vi "User scan tool box.vi"() -> ()   [LabVIEW 2021]
doc: "This example demonstrates how you can create your own \"toolbox\": a custom designed VI that regroups all the controls you want to access quickly.\n\nThis example displays the most used controls to perform STM scanning (current, bias, gain, scan frame, tilt).\n\n- Nanonis Programming Interface -"
uses:
  Nanonis Prog Interface.lvlib
panel:
  out "Status":bool
  in  "stop":bool
  in  "Bias (V)":sgl=0.5 min=-10 max=10 format="%_4p"
  in  "Speed":sgl(slide)=1.0 caption="Time per line (s)" min=0.01 max=10 scale=0.01..2.0 scale format="%.0p"
  in  "Current (A)":sgl=1e-09 format="%_4p"
  in  "Scan":bool
  in  "Images basename":string="SampleTest_"
  in  "Tilt Y (deg)":sgl min=-30 max=30 format="%.3f"
  in  "Tilt X (deg)":sgl min=-30 max=30 format="%.3f"
  in  "Position Yc":sgl min=-1e-05 max=1e-05 format="%.2p"
  in  "Position Xc":sgl min=-1e-05 max=1e-05 format="%.2p"
  in  "Height (m)":sgl=1e-07 min=1e-12 max=1e-05 format="%#.2p"
  in  "Width (m)":sgl=1e-07 min=1e-12 max=1e-05 format="%#.2p"
  in  "Angle (deg)":sgl format="%.2f"
  in  "P-gain":sgl(slide)=1e-10 scale=1e-11..1e-08 scale format="%.0p"
  in  "Lines":i32=256 min=1 max=2048
  in  "Pixels":i32=256 min=16 max=2048
  # "Scan parameters"
  # "Scan frame"
  # "Correction"
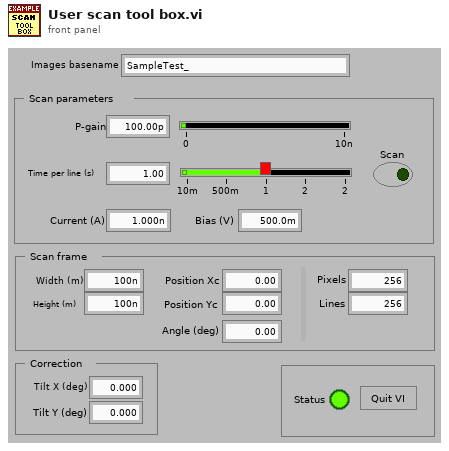
[diagram p1: front panel]
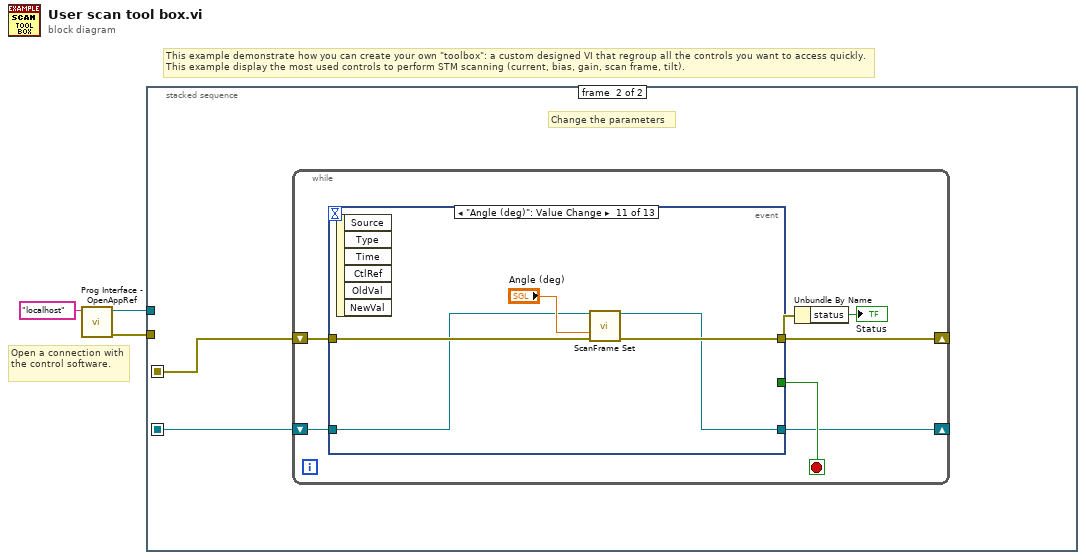
[diagram p0: block diagram]
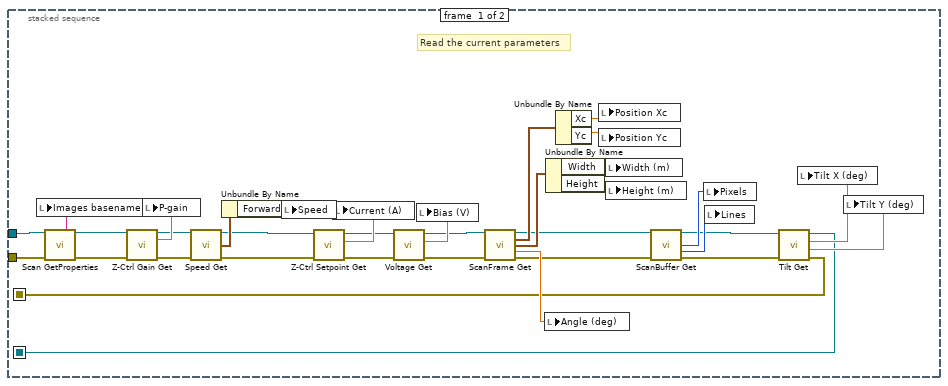
[diagram p2: hidden frame]
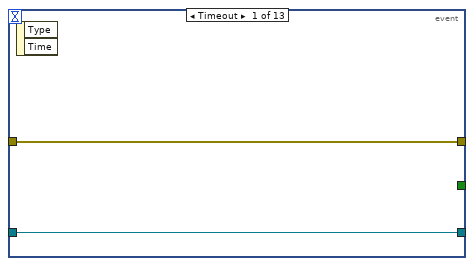
[diagram p3: hidden frame]
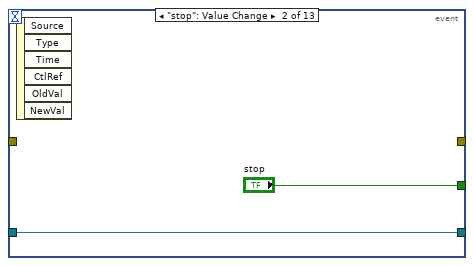
[diagram p4: hidden frame]
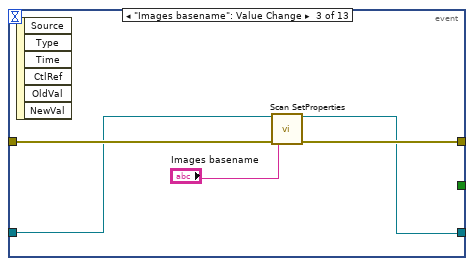
[diagram p5: hidden frame]
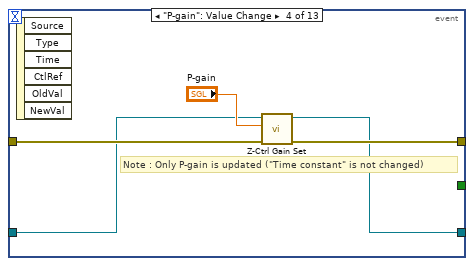
[diagram p6: hidden frame]
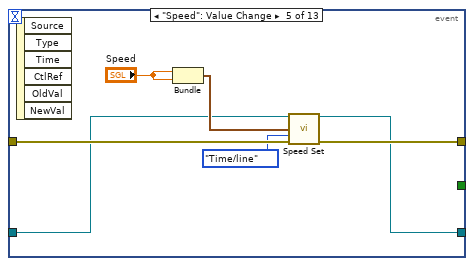
[diagram p7: hidden frame]
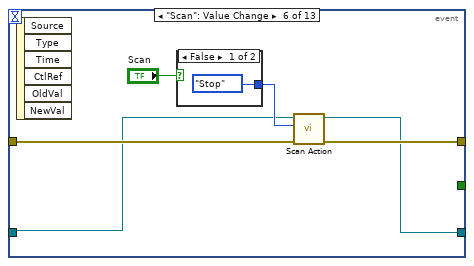
[diagram p8: hidden frame]
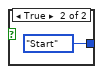
[diagram p9: hidden frame]
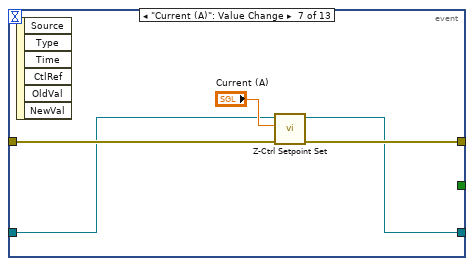
[diagram p10: hidden frame]
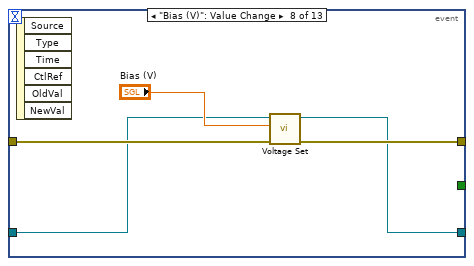
[diagram p11: hidden frame]
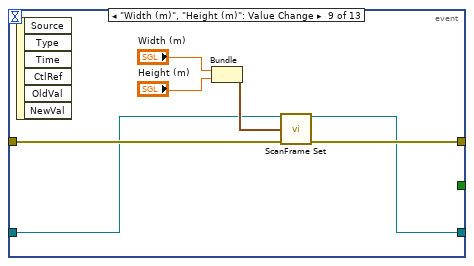
[diagram p12: hidden frame]
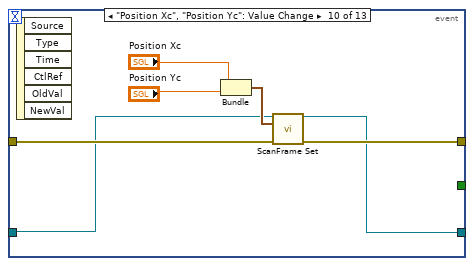
[diagram p13: hidden frame]
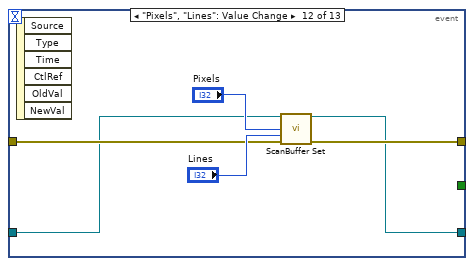
[diagram p14: hidden frame]
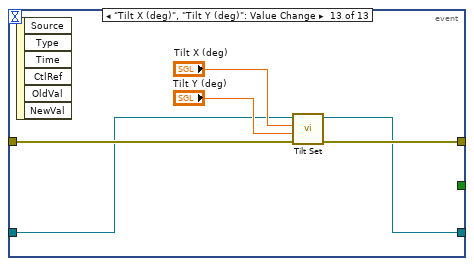
[diagram p15: hidden frame]
diagram:
  # "Open a connection with the control software."
  # "This example demonstrate how you can create your own \"toolbox\": a custom designed VI that regroup all the controls you want to access quickly.\nThis example display the most used controls to perform STM scanning (current, bias, gain, scan frame, tilt)."
  n1 = call <userlib>:"Prog Interface - OpenAppRef.vi"("Machine name (local machine IP)"="localhost" ("Machine name (localhost)")) -> ("Error out"=w2:errorcluster, "Application reference"=w1:refnum<vi>)  [unwired: 5 in]
  n2 = stacked-sequence {
    seq-local: [w19 _] -> [_ w40]
    seq-local: [w4 _] -> [_ w39]
    tunnel: w2 -> [w18 _]
    tunnel: w1 -> [w15 _]
    frame #0 {
      # "Read the current parameters"
      n3 = call <userlib>:"Scan GetProperties.vi"("Application ref in"=w15, "Error in (no error)"=w18) -> ("Application ref out"=w14:refnum<vi>, "Serie name"=w16:string, "Error out"=w17:errorcluster)  [unwired: 6 in, 5 out]
      n4 = local write "Images basename"(w16) -> ()
      n5 = call <userlib>:"Z-Ctrl Gain Get.vi"("Application ref in"=w14, "error in (no error)"=w17) -> ("Application ref out"=w13:refnum<vi>, "P-gain"=w38:sgl, "error out"=w37:errorcluster)  [unwired: 9 in, 2 out]
      n6 = local write "P-gain"(w38) -> ()
      n7 = call <userlib>:"Speed Get.vi"("Application ref in"=w13, "error in (no error)"=w37) -> ("Application ref out"=w12:refnum<vi>, "Time/line (s)"=w36:cluster{"Forward":sgl, "Backward":sgl}, "error out"=w34:errorcluster)  [unwired: 8 in, 3 out]
      n8 = Unbundle By Name(w36) -> ("Forward"=w35:sgl)
      n9 = local write "Speed"(w35) -> ()
      n10 = call <userlib>:"Z-Ctrl Setpoint Get.vi"("error in (no error)"=w34, "Application ref in"=w12) -> ("error out"=w33:errorcluster, "Z Controller setpoint"=w11:sgl, "Application ref out"=w10:refnum<vi>)  [unwired: 6 in]
      n11 = local write "Current (A)"(w11) -> ()
      n12 = call <userlib>:"Voltage Get.vi"("error in (no error)"=w33, "Application ref in"=w10) -> ("error out"=w31:errorcluster, "Bias (V)"=w32:sgl, "Application ref out"=w9:refnum<vi>)  [unwired: 7 in]
      n13 = local write "Bias (V)"(w32) -> ()
      n14 = call <userlib>:"ScanFrame Get.vi"("Application ref in"=w9, "error in (no error)"=w31) -> ("Application ref out"=w8:refnum<vi>, "Center coordinates (m)"=w30:cluster{"Xc":sgl, "Yc":sgl}, "Size (m)"=w29:cluster{"Width":sgl, "Height":sgl}, "Angle (deg)"=w28:sgl, "error out"=w23:errorcluster)  [unwired: 9 in]
      n15 = local write "Angle (deg)"(w28) -> ()
      n16 = Unbundle By Name(w29) -> ("Width"=w25:sgl, "Height"=w24:sgl)
      n17 = Unbundle By Name(w30) -> ("Xc"=w27:sgl, "Yc"=w26:sgl)
      n18 = local write "Position Xc"(w27) -> ()
      n19 = local write "Position Yc"(w26) -> ()
      n20 = local write "Width (m)"(w25) -> ()
      n21 = local write "Height (m)"(w24) -> ()
      n22 = call <userlib>:"ScanBuffer Get.vi"("Application ref in"=w8, "error in (no error)"=w23) -> ("Application ref out"=w5:refnum<vi>, "Pixels/line"=w22:i32, "Lines"=w21:i32, "error out"=w20:errorcluster)  [unwired: 9 in, 1 out]
      n23 = local write "Pixels"(w22) -> ()
      n24 = local write "Lines"(w21) -> ()
      n25 = call <userlib>:"Tilt Get.vi"("error in (no error)"=w20, "Application ref in"=w5) -> ("error out"=w19:errorcluster, "Tilt Y (deg)"=w7:sgl, "Tilt X (deg)"=w6:sgl, "Application ref out"=w4:refnum<vi>)  [unwired: 6 in]
      n26 = local write "Tilt X (deg)"(w6) -> ()
      n27 = local write "Tilt Y (deg)"(w7) -> ()
    }
    frame #1 {
      # "Change the parameters"
      n28 = while {
        shift-right: [w44] -> _
        shift-left: w40 -> [w46]
        shift-right: [w41] -> _
        shift-left: w39 -> [w42]
        stop <- w45 stop-if-true
        n29 = event shown="[10] \"Angle (deg)\": Value Change" {
          selector: _ -> [_ _ _ _ _ _ _ _ _ _ _ _ _]
          dyn-events: _ -> [_ _ _ _ _ _ _ _ _ _ _ _ _]
          timeout: _ -> [_ _ _ _ _ _ _ _ _ _ _ _ _]
          tunnel: w46 -> [w48 _ w55 w60 w67 w73 w79 w84 w89 w99 w104 w108 w116]
          tunnel: [w48 _ w54 w59 w66 w72 w78 w83 w88 w98 w103 w107 w115] -> w44
          tunnel: [_ "stop" _ _ _ _ _ _ _ _ _ _ _] -> w45
          tunnel: [w47 w49 w51 w56 w61 w68 w76 w81 w86 w93 w100 w105 w111] -> w41
          tunnel: w42 -> [w47 w49 w52 w57 w62 w69 w77 w82 w87 w94 w101 w106 w112]
          event Timeout {
            n30 = event-data() -> ()  [unwired: 1 in, 2 out]
          }
          event "stop": Value Change {
            n31 = event-data() -> ()  [unwired: 1 in, 6 out]
          }
          event "Images basename": Value Change {
            n32 = event-data() -> ()  [unwired: 1 in, 6 out]
            n33 = call <userlib>:"Scan SetProperties.vi"("Application ref in"=w52, "Error in (no error)"=w55, "Serie name"="Images basename") -> ("Application ref out"=w51:refnum<vi>, "Error out"=w54:errorcluster)  [unwired: 11 in]
          }
          event "P-gain": Value Change {
            # "Note : Only P-gain is updated (\"Time constant\" is not changed)"
            n34 = event-data() -> ()  [unwired: 1 in, 6 out]
            n35 = call <userlib>:"Z-Ctrl Gain Set.vi"("error in (no error)"=w60, "P-gain"="P-gain", "Application ref in"=w57) -> ("error out"=w59:errorcluster, "Application ref out"=w56:refnum<vi>)  [unwired: 6 in]
          }
          event "Speed": Value Change {
            n36 = event-data() -> ()  [unwired: 1 in, 6 out]
            n37 = Bundle("Speed"="Speed", "Speed"="Speed") -> (w64:cluster{"Speed":sgl, "Speed":sgl})  [unwired: 1 in]
            n38 = call <userlib>:"Speed Set.vi"("Application ref in"=w62, "Time/line (s)"=w64, "Keep constant"=enum16{"No change", "Speed", "Time/line"}."Time/line", "error in (no error)"=w67) -> ("Application ref out"=w61:refnum<vi>, "error out"=w66:errorcluster)  [unwired: 10 in]
          }
          event "Scan": Value Change {
            n39 = event-data() -> ()  [unwired: 1 in, 6 out]
            n40 = case shown="False" "Scan" {
              tunnel: [enum16{"Start", "Stop", "Pause", "Resume"}."Stop" ("Scan action") enum16{"Start", "Stop", "Pause", "Resume"}."Start" ("Scan action")] -> w70
              frame False {
              }
              frame True {
              }
            }
            n41 = call <userlib>:"Scan Action.vi"("error in (no error)"=w73, "Scan action (Start)"=w70, "Application ref in"=w69) -> ("error out"=w72:errorcluster, "Application ref out"=w68:refnum<vi>)  [unwired: 6 in]
          }
          event "Current (A)": Value Change {
            n42 = event-data() -> ()  [unwired: 1 in, 6 out]
            n43 = call <userlib>:"Z-Ctrl Setpoint Set.vi"("error in (no error)"=w79, "Z Controller setpoint"="Current (A)", "Application ref in"=w77) -> ("error out"=w78:errorcluster, "Application ref out"=w76:refnum<vi>)  [unwired: 7 in]
          }
          event "Bias (V)": Value Change {
            n44 = event-data() -> ()  [unwired: 1 in, 6 out]
            n45 = call <userlib>:"Voltage Set.vi"("Error in (no error)"=w84, "Bias (V)"="Bias (V)", "Application ref in"=w82) -> ("Error out"=w83:errorcluster, "Application ref out"=w81:refnum<vi>)  [unwired: 7 in]
          }
          event "Width (m)", "Height (m)": Value Change {
            n46 = event-data() -> ()  [unwired: 1 in, 6 out]
            n47 = Bundle("Width (m)"="Width (m)", "Height (m)"="Height (m)") -> (w90:cluster{"Width (m)":sgl, "Height (m)":sgl})  [unwired: 1 in]
            n48 = call <userlib>:"ScanFrame Set.vi"("Application ref in"=w87, "Size (m)"=w90, "error in (no error)"=w89) -> ("Application ref out"=w86:refnum<vi>, "error out"=w88:errorcluster)  [unwired: 11 in]
          }
          event "Position Xc", "Position Yc": Value Change {
            n49 = event-data() -> ()  [unwired: 1 in, 6 out]
            n50 = Bundle("Position Xc"="Position Xc", "Position Yc"="Position Yc") -> (w95:cluster{"Position Xc":sgl, "Position Yc":sgl})  [unwired: 1 in]
            n51 = call <userlib>:"ScanFrame Set.vi"("Application ref in"=w94, "Center coordinates (m)"=w95, "error in (no error)"=w99) -> ("Application ref out"=w93:refnum<vi>, "error out"=w98:errorcluster)  [unwired: 11 in]
          }
          event "Angle (deg)": Value Change {
            n52 = event-data() -> ()  [unwired: 1 in, 6 out]
            n53 = call <userlib>:"ScanFrame Set.vi"("Application ref in"=w101, "Angle (deg)"="Angle (deg)", "error in (no error)"=w104) -> ("Application ref out"=w100:refnum<vi>, "error out"=w103:errorcluster)  [unwired: 11 in]
          }
          event "Pixels", "Lines": Value Change {
            n54 = event-data() -> ()  [unwired: 1 in, 6 out]
            n55 = call <userlib>:"ScanBuffer Set.vi"("Application ref in"=w106, "Pixels"="Pixels", "Lines"="Lines", "error in (no error)"=w108) -> ("Application ref out"=w105:refnum<vi>, "error out"=w107:errorcluster)  [unwired: 10 in]
          }
          event "Tilt X (deg)", "Tilt Y (deg)": Value Change {
            n56 = event-data() -> ()  [unwired: 1 in, 6 out]
            n57 = call <userlib>:"Tilt Set.vi"("error in (no error)"=w116, "Tilt Y (deg)"="Tilt Y (deg)", "Tilt X (deg)"="Tilt X (deg)", "Application ref in"=w112) -> ("error out"=w115:errorcluster, "Application ref out"=w111:refnum<vi>)  [unwired: 6 in]
          }
        }
        n58 = Unbundle By Name(w44) -> ("status"=→"Status":bool)
      }
    }
  }
